vi "ActionVIOnLoad.vi"(8 "error in (no error)":errorcluster, 11 "Device Item Ref in":T1 format="%.0x") -> (0 "error out":errorcluster, 3 "Device Item Ref out":T1 format="%.0x")   [LabVIEW 2020, in "Ballard ARINC 429 System Explorer.lvlib"]
uses:
  Ballard ARINC 429 System Explorer.lvlib
  <vilib>/NI VeriStand/Custom Device API/Custom Device Item Ref.ctl
  Includes/Ballard ARINC 429 System Explorer.lvlibp/Custom Device Support/System Explorer/Implementation/Implementation.lvlib
  <vilib>/NI VeriStand/Custom Device API/Custom Device API.lvlib
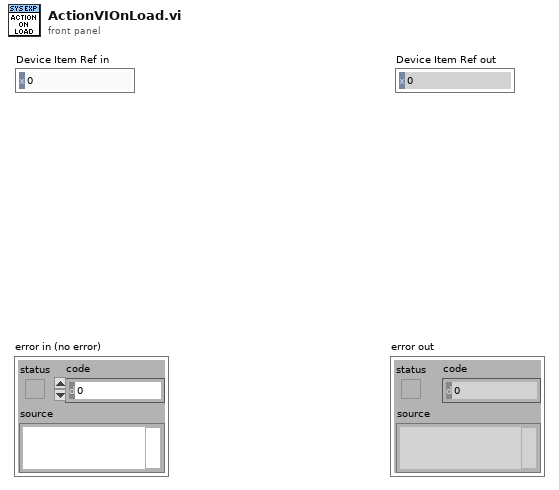
[diagram p1: front panel]
types:
  T1 = typedef "Custom Device API.lvlib/Custom Device Item Ref.ctl" = u64
  T2 = typedef "Ballard ARINC 429 System Explorer.lvlibp/Custom Device API.lvlib/Custom Device Item Ref.ctl" = u64
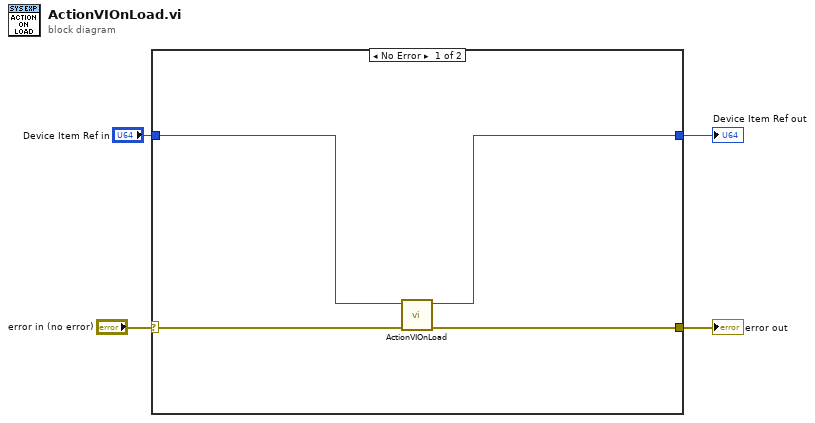
[diagram p0: block diagram]
diagram:
  n1 = case shown="No Error" "error in (no error)" {
    selector: "error in (no error)" -> [w8 w10]
    tunnel: [w7 w10] -> w3
    tunnel: "Device Item Ref in" -> [w5 w9]
    tunnel: [w6 w9] -> w1
    frame No Error {
      n2 = call "ActionVIOnLoad.vi"("error in"=w8, "Device Item Ref"=w5) -> ("error out"=w7:errorcluster, "Device Item Ref out"=w6:T2)  [unwired: 8 in]
    }
    frame Error {
    }
  }
  "error out" <- w3
  "Device Item Ref out" <- w1
